vi "SetSampleCount.vi"(8 "error in (no error)":errorcluster caption="错误输入（无错误）", 11 "XYPlot 输入":refnum<class "TrendPlot.lvclass">) -> (0 "error out":errorcluster caption="错误输出", 3 "XYPlot 输出":refnum<class "TrendPlot.lvclass">)   [LabVIEW 2018, in "DataDisplay.lvlib" / "TrendPlot.lvclass"]
uses:
  TrendPlot.lvclass
  TypeDefine/DD_Command.ctl
  TrendPlot.lvclass/TrendPlot.ctl
  DataDisplay.lvlib
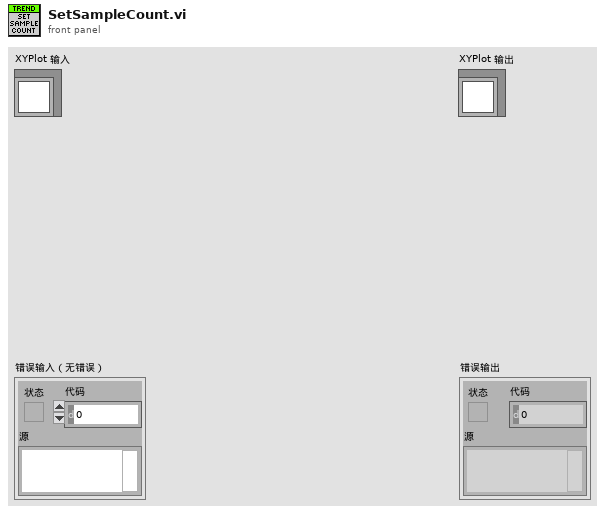
[diagram p1: front panel]
types:
  T1 = typedef "DataDisplay.lvlib/DD_Command.ctl" = cluster{"消息":string, "参数":variant}
  T2 = typedef "DataDisplay.lvlib/DD_CommandQ.ctl" = refnum<queue>
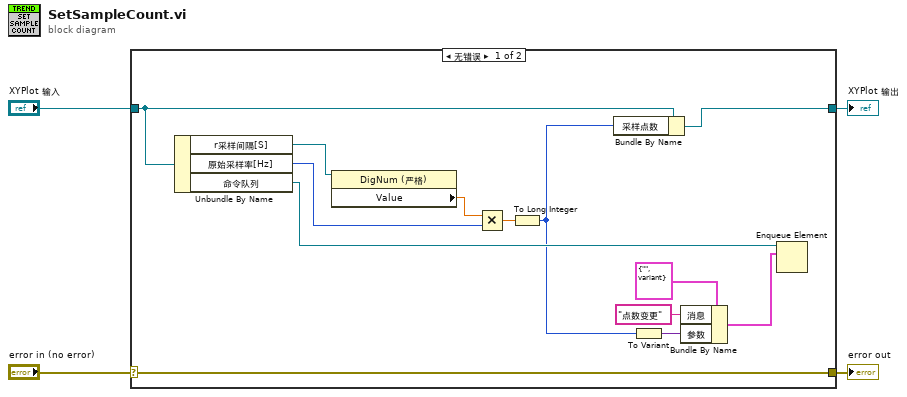
[diagram p0: block diagram]
diagram:
  n1 = case shown="无错误" "error in (no error)" {
    selector: "error in (no error)" -> [w17 w19]
    tunnel: [w17 w19] -> w3
    tunnel: [w11 w18] -> w1
    tunnel: "XYPlot 输入" -> [w16 w18]
    frame No Error {
      n2 = Unbundle By Name(w16) -> ("r采样间隔[S]"=w12:refnum<vi>, "原始采样率[Hz]"=w13:i32, "命令队列"=w10:T2)
      n3 = property class="DigNum (严格)"(reference=w12) -> ("Value"=w15:dbl)  [unwired: 1 in, 2 out]
      n4 = Multiply(x=w15, y=w13) -> (x*y=w14:dbl)
      n5 = To Long Integer(number=w14) -> (32bit integer=w6:i32)
      n6 = Bundle By Name(cluster=w16, "采样点数"=w6) -> (w11:refnum<class "TrendPlot.lvclass">)
      n7 = To Variant(anything=w6) -> (Variant=w5:variant)
      n8 = Bundle By Name(cluster=T1 {"消息"="", "参数"=variant} ("命令"), "消息"="点数变更", "参数"=w5) -> (w7:T1)
      n9 = Enqueue Element(queue=w10, element=w7) -> ()  [unwired: 2 in, 3 out]
    }
    frame Error {
    }
  }
  "error out" <- w3
  "XYPlot 输出" <- w1
